vi "Configure Onboard Clock.vi"(0 "device session in":refnum<class "Device Session.lvclass">, 5 "reference clock source":T1, 7 "reference clock rate (Hz)":dbl=250000000.0 format="%#_6p", 11 "error in":errorcluster) -> (4 "device session out":refnum<class "Device Session.lvclass">, 6 "actual adc clock rate (Hz)":dbl=250000000.0 format="%#_6p", 8 "actual reference clock rate (Hz)":dbl format="%#_6p", 15 "error out":errorcluster)   [LabVIEW 2015, in "Device Session.lvclass"]
doc: "Configures the device to use an onboard clock as the source of the ADC clock. If a reference clock source is specified, this VI also phase locks the device to that clock.\n\n<B>Input Parameters</B>\n\n<B>device session in</B> is a reference to the session containing sessions to all instrument design libraries used in this sample project. This parameter is obtained from the 'Open Session' VI.\n\n<B>reference clock source</B> specifies the source of the reference clock used to generate the onboard ADC Clock.\n\n'None' (default): specifies that no reference clock will be used.\n'Clock In': specifies that the clock source is the Clock In connector on the device front panel.\n'PXI Clock': specifies that the clock source is the clock signal from the PXI chassis.\n\n<B>reference clock rate (Hz)</B> specifies the input reference clock rate if the 'reference clock source' is Clock In. This parameter is ignored if the 'reference clock source' is None or PXI Clock.\n\n<B>error in</B> describes error conditions that occur before this node runs. This input provides standard 'error in' functionality.\n\n<B>Output Parameters</B>\n\n<B>device session out</B> passes a reference to the session to the next VI.\n\n<B>actual adc clock rate (Hz)</B> returns the coerced value of the ADC clock rate.\n\n<B>actual reference clock rate (Hz)</B> returns the coerced reference clock rate.\n\n<B>error out</B> contains error information. This output provides standard 'error out' functionality."
uses:
  Device Session.lvclass
  <instrlib>/HSAI-RIO/Types/v1/Host/Typedefs/Reference Clock Source.ctl
  Device Session.lvclass/Device Session.ctl
  <instrlib>/HSAI-RIO/Config/Interface/v1/Host/Protected/Configure ADC Clock For Onboard.vi
  <instrlib>/HSAI-RIO/Config/Interface/v1/Host/niHSAI Config v1 Host.lvclass
  <instrlib>/HSAI-RIO/Types/v1/Host/niHSAI Types v1 Host.lvlib
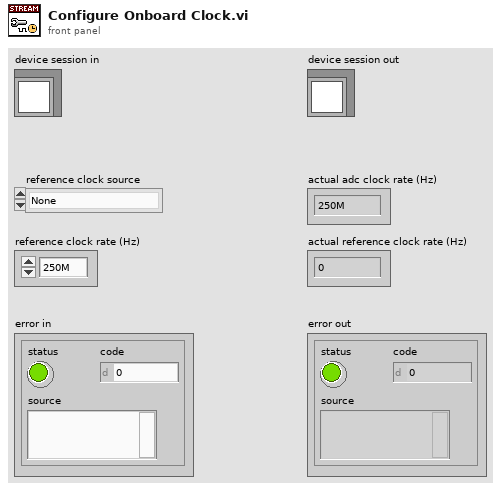
[diagram p1: front panel]
types:
  T1 = typedef "niHSAI Types v1 Host.lvlib/Reference Clock Source.ctl" = enum8{"None", "Clock In", "PXI Clock"}
  T2 = typedef "Device Session.lvclass/Device Session Object.ctl" = cluster{"ni5171R FPGA Reference":T3, "niHSAI config":refnum<class "niHSAI Config v1 Host.lvclass">, "configured scaling coefficients":cluster{"gain":dbl, "offset":dbl}[], "number of channels to stream":u8, "selected acq channels":bool[], "number of channels":u32, "actual channel configuration":T4[], "configured channels":bool[], "sample clock rate (Hz)":dbl}
  T3 = typedef "Device Session.lvclass/FPGA Refnum.ctl" = refnum<k20>
  T4 = typedef "niHSAI Types v1 Host.lvlib/Channel Configuration.ctl" = cluster{"channel":u32, "coupling":T5, "impedance":T6, "bandwidth":T7, "vertical range":dbl, "vertical offset":dbl}
  T5 = typedef "niHSAI Types v1 Host.lvlib/Coupling.ctl" = enum8{"Default", "DC", "AC"}
  T6 = typedef "niHSAI Types v1 Host.lvlib/Impedance.ctl" = enum8{"Default", "1 mega ohm", "50 ohm"}
  T7 = typedef "niHSAI Types v1 Host.lvlib/Bandwidth.ctl" = enum8{"Default", "Full Bandwidth", "Anti-alias Filter"}
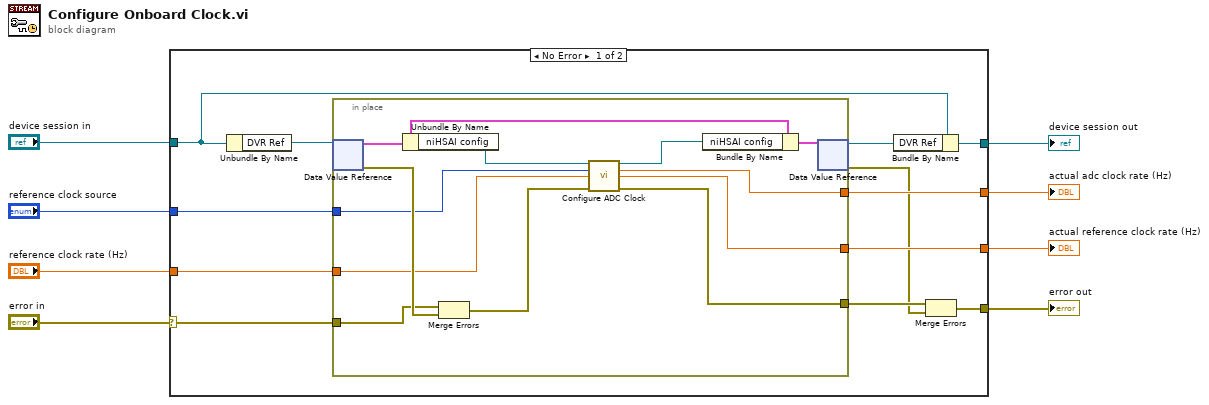
[diagram p0: block diagram]
diagram:
  n1 = case shown="No Error" "error in" {
    selector: "error in" -> [w20 w34]
    tunnel: "device session in" -> [w15 w33]
    tunnel: [w14 w33] -> w6
    tunnel: [w17 w34] -> w5
    tunnel: [w19 _] -> w2
    tunnel: [w13 _] -> w1
    tunnel: "reference clock source" -> [w12 _]
    tunnel: "reference clock rate (Hz)" -> [w11 _]
    frame No Error {
      n2 = Unbundle By Name(w15) -> ("DVR Ref"=w16:refnum<data-value>)
      n3 = in-place {
        in-place-border: w20 -> [w21]
        in-place-border: [w32] -> w19
        in-place-border: [w31] -> w10
        in-place-border: [w24] -> w13
        in-place-border: w12 -> [w23]
        in-place-border: w11 -> [w22]
        n4 = in-place-dvr #1(w16) -> (w25:T2, w29:errorcluster)
        n5 = Unbundle By Name(w25) -> ("niHSAI config"=w27:refnum<class "niHSAI Config v1 Host.lvclass">)
        n6 = Merge Errors(w21, w29) -> (w28:errorcluster)
        n7 = call-poly <instrlib>:"Configure ADC Clock.vi"("session in"=w27, "reference clock source"=w23, "reference clock rate (Hz)"=w22, "error in"=w28) -> ("session out"=w30:refnum<class "niHSAI Config v1 Host.lvclass">, "actual adc clock rate (Hz)"=w32:dbl, "fpga data clock rate (Hz)"=w24:dbl, "error out"=w31:errorcluster)  [unwired: 7 in, 1 out]
        n8 = Bundle By Name(cluster=w25, "niHSAI config"=w30) -> (w26:T2)
        n9 = in-place-dvr #1(w26) -> (w18:refnum<data-value>, w9:errorcluster)
      }
      n10 = Bundle By Name(cluster=w15, "DVR Ref"=w18) -> (w14:refnum<class "Device Session.lvclass">)
      n11 = Merge Errors(w10, w9) -> (w17:errorcluster)
    }
    frame Error {
    }
  }
  "error out" <- w5
  "device session out" <- w6
  "actual adc clock rate (Hz)" <- w2
  "actual reference clock rate (Hz)" <- w1
